vi "To String.vi"(8 "error in (no error)":errorcluster, 11 "Semver in":refnum<class "Semver.lvclass">) -> (0 "error out":errorcluster, 2 "Version String":string)   [LabVIEW 2017, in "Semver.lvlib" / "Semver.lvclass"]
uses:
  Semver.lvclass
  Semver.lvclass/Semver.ctl
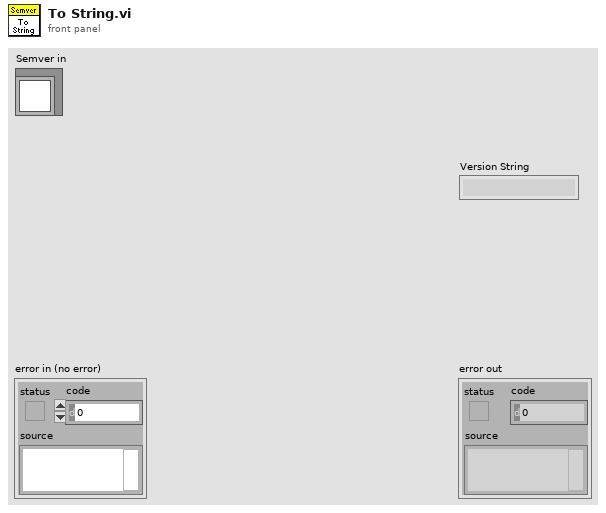
[diagram p1: front panel]
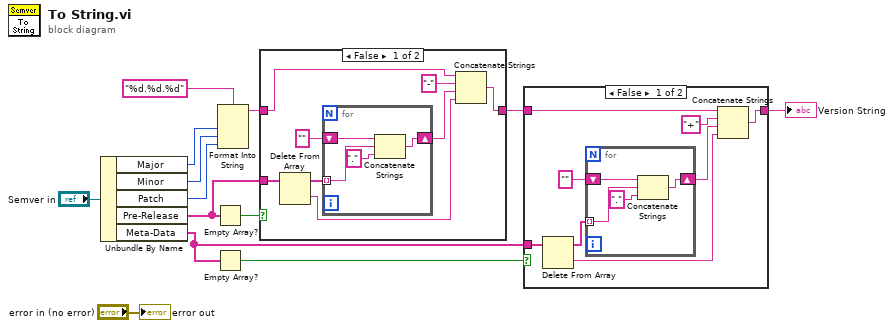
[diagram p0: block diagram]
diagram:
  n1 = Unbundle By Name("Semver in") -> ("Major"=w11:i32, "Minor"=w10:i32, "Patch"=w9:i32, "Pre-Release"=w5:string[], "Meta-Data"=w2:string[])
  n2 = Empty Array?(array=w5) -> (empty?=w6:bool)
  n3 = Empty Array?(array=w2) -> (empty?=w3:bool)
  n4 = Format Into String(format string="%d.%d.%d", w11, w10, w9) -> (resulting string=w7:string)  [unwired: 2 in, 1 out]
  n5 = case shown="False" w6 {
    tunnel: [w20 w26] -> w4
    tunnel: w7 -> [w21 w26]
    tunnel: w5 -> [w18 _]
    frame False {
      n6 = Delete From Array(array=w18) -> (deleted portion=w14:string, array with subset deleted=w15:string[])  [unwired: 2 in]
      n7 = for {
        tunnel: w15 -> [w25] mode=indexing
        shift-right: [w24] -> w16
        shift-left: "" -> [w23]
        n8 = Concatenate Strings(w23, w25, ".") -> (w24:string)
      }
      n9 = Concatenate Strings(w21, "-" ("string"), w16, w14) -> (w20:string)
    }
    frame True {
    }
  }
  n10 = case shown="False" w3 {
    tunnel: [w33 w39] -> w1
    tunnel: w4 -> [w34 w39]
    tunnel: w2 -> [w31 _]
    frame False {
      n11 = Delete From Array(array=w31) -> (deleted portion=w27:string, array with subset deleted=w28:string[])  [unwired: 2 in]
      n12 = for {
        tunnel: w28 -> [w38] mode=indexing
        shift-right: [w37] -> w29
        shift-left: "" -> [w36]
        n13 = Concatenate Strings(w36, w38, ".") -> (w37:string)
      }
      n14 = Concatenate Strings(w34, "+" ("string"), w29, w27) -> (w33:string)
    }
    frame True {
    }
  }
  "Version String" <- w1
  "error out" <- "error in (no error)"
